vi "Test Query Parameters.vi"() -> ()   [LabVIEW 2020]
uses:
  HTTP Server/Trace Log.ctl
  HTTP Server/Trace Item.ctl
  HTTP Server/Processing Step.ctl
  <vilib>/IlluminatedG/IG HTTP Utils/HTTP Utils/Method.ctl
  TestQueryParamController/TestQueryParamController.lvclass
  C:/dev/illuminated-g/lv-http-server/HTTP Server/Handler/Handler.lvclass
  HTTP Server/Server/Add Connection Handler.vi
  HTTP Server/Server/Add Request Handler.vi
  HTTP Server/Server/Add Route Handler.vi
  HTTP Server/Server/Add Controller Handler.vi
  HTTP Server/Server/Add Controller.vi
  HTTP Server/Server/Add Response Handler.vi
  HTTP Server/Server/Add Complete Handler.vi
  HTTP Server/Server/Add Exception Handler.vi
  HTTP Server/Connection Handler/Connection Handler.lvclass
  HTTP Server/Request Handler/Request Handler.lvclass
  HTTP Server/Route Handler/Route Handler.lvclass
  HTTP Server/Controller Handler/Controller Handler.lvclass
  HTTP Server/Controller/Controller.lvclass
  HTTP Server/Response Handler/Response Handler.lvclass
  HTTP Server/Complete Handler/Complete Handler.lvclass
  HTTP Server/Exception Handler/Exception Handler.lvclass
  HTTP Server/Server/Server.lvclass
  HTTP Server/Handler/Handler.lvclass
  HTTP Server/RequestTraceLog/RequestTraceLog.lvclass
  HTTP Server/HTTP Server.lvlib
  <vilib>/IlluminatedG/IG HTTP Utils/HTTP Utils/HTTP Utils.lvlib
panel:
  out "error out":errorcluster
  in  "Refresh Traces":bool
  out "Traces":T1[](array[typedef])=[{"Items"=[{"Duration"=0.00019280000014987309, "Step"=enum."Connection", "Class"="", "Info"="Start Request Parsing", "Status"=FALSE, "Code"=0, "Time"=3234.2736639}, {"Duration"=104.21120999999994, "Step"=enum."Connection", "Class"="", "Info"="Request Initialized", "Status"=TRUE, "Code"=66, "Time"=3338.4848739}, {"Duration"=0.0007422999997288571, "Step"=enum."Connection", "Class"="HTTP Utils.lvlib:Response.lvclass", "Info"="Completed", "Status"=TRUE, "Code"=66, "Time"=3338.4856161999996}], "Client"="tcp://DAB-2020SP1x86.ni.corp.natinst.com:52788", "Target"="", "Response Type"="", "Processing"=0.0007728000000497559, "Status"=200, "Method"=enum."GET", "Content Type"="", "Request Headers"=[], "Parsing"=3338.4848739, "Waiting"=-3234.2736639, "Identity"="", "Loaded"=FALSE, "Created"=FALSE, "Destroyed"=FALSE, "Response Headers"=[], "Created"=0.0, "Expires"=0.0, "Roles"=[], "Sending"=0.0}, {"Items"=[{"Duration"=0.006463199999870994, "Step"=enum."Connection", "Class"="", "Info"="Start Request Parsing", "Status"=FALSE, "Code"=0, "Time"=3459.3199179}, {"Duration"=0.008297200000015437, "Step"=enum."Connection", "Class"="", "Info"="Request Initialized", "Status"=TRUE, "Code"=66, "Time"=3459.3282151}, {"Duration"=0.0001554000000396627, "Step"=enum."Connection", "Class"="HTTP Utils.lvlib:Response.lvclass", "Info"="Completed", "Status"=TRUE, "Code"=66, "Time"=3459.3283705}], "Client"="tcp://DAB-2020SP1x86.ni.corp.natinst.com:52995", "Target"="", "Response Type"="", "Processing"=0.00019930000007661874, "Status"=200, "Method"=enum."GET", "Content Type"="", "Request Headers"=[], "Parsing"=3459.3282151, "Waiting"=-3459.3199179, "Identity"="", "Loaded"=FALSE, "Created"=FALSE, "Destroyed"=FALSE, "Response Headers"=[], "Created"=0.0, "Expires"=0.0, "Roles"=[], "Sending"=0.0}] {"Sending" format="%_6f"; "Expires" format="%<%X %x>T"; "Created" format="%<%X %x>T"; "Waiting" format="%_6f"; "Parsing" format="%_6f"; "Processing" format="%_6f"; "Items"."Time" format="%.6f"; "Items"."Duration" format="%.6f"}
  in  "Port":u16=36987
  # "This can be viewed at http://localhost:36987/calc and filling out the query parameters as specified in the page.\n\nRequests to any other path will result in a 404 status."
  # "Request"
  # "Response"
  # "Session"
  # "Auth"
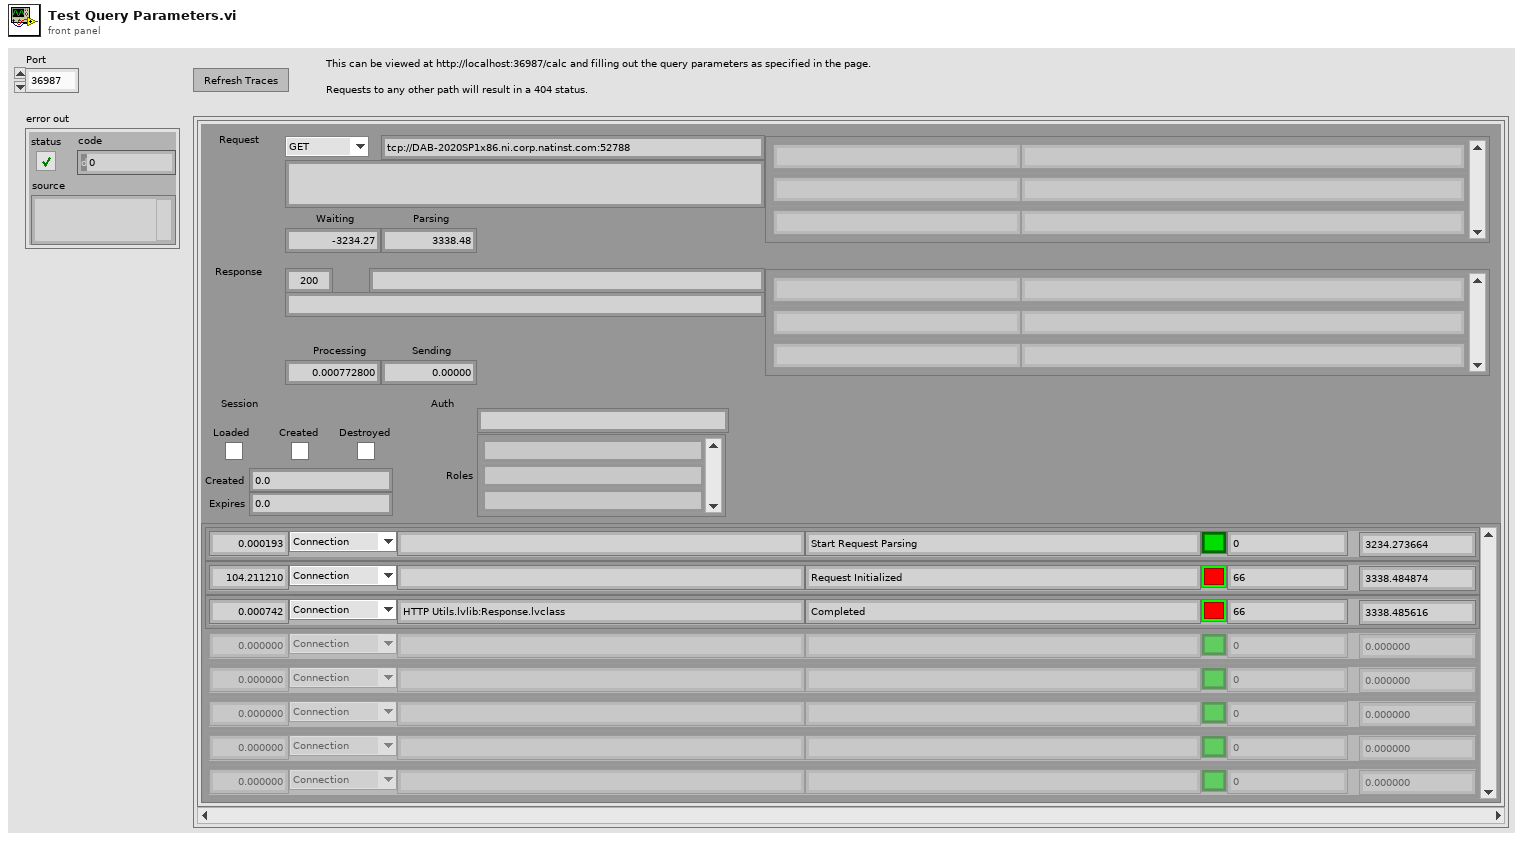
[diagram p1: front panel]
types:
  T1 = typedef "HTTP Server.lvlib/Trace Log.ctl" = cluster{"Items":T2[], "Client":string, "Target":string, "Response Type":string, "Processing":dbl, "Status":u16, "Method":T4, "Content Type":string, "Request Headers":cluster{"Name":string, "Value":string}[], "Parsing":dbl, "Waiting":dbl, "Identity":string, "Loaded":bool, "Created":bool, "Destroyed":bool, "Response Headers":cluster{"Name":string, "Value":string}[], "Created":dbl, "Expires":dbl, "Roles":string[], "Sending":dbl}
  T2 = typedef "HTTP Server.lvlib/Trace Item.ctl" = cluster{"Duration":dbl, "Step":T3, "Class":string, "Info":string, "Status":bool, "Code":i32, "Time":dbl}
  T3 = typedef "HTTP Server.lvlib/Processing Step.ctl" = enum16{"Connection", "Request", "Routing", "Controller Init", "Controller", "Response", "Complete", "Exception"}
  T4 = typedef "HTTP Utils.lvlib/Method.ctl" = enum16{"GET", "HEAD", "POST", "PUT", "DELETE", "CONNECT", "OPTIONS", "TRACE", "PATCH"}
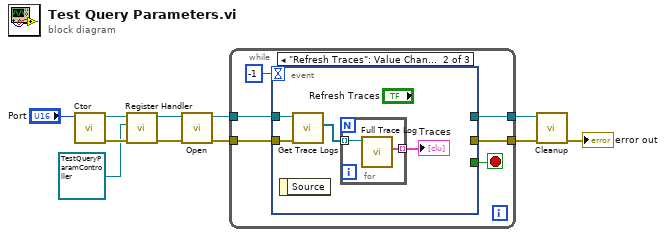
[diagram p0: block diagram]
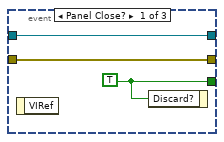
[diagram p2: hidden frame]
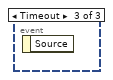
[diagram p3: hidden frame]
diagram:
  n1 = call "Ctor.vi"("HTTP Port (80)"="Port") -> ("error out"=w3:errorcluster, "Server out"=w6:refnum<class "Server.lvclass">)  [unwired: 9 in]
  n2 = call "Register Handler.vi"("error in (no error)"=w3, "Handler"=refnum<class "TestQueryParamController.lvclass"> refnum ("TestQueryParamController.lvclass"), "Server in"=w6) -> ("error out"=w4:errorcluster, "Server out"=w5:refnum<class "Server.lvclass">)  [unwired: 7 in]
  n3 = call "Open.vi"("error in (no error)"=w4, "Server in"=w5) -> ("error out"=w9:errorcluster, "Server out"=w10:refnum<class "Server.lvclass">)  [unwired: 8 in]
  n4 = while {
    tunnel: w10 -> [w15]
    tunnel: w9 -> [w16]
    tunnel: [w14] -> w8
    tunnel: [w13] -> w7
    stop <- w17 stop-if-true
    n5 = event shown="[1] \"Refresh Traces\": Value Change" {
      selector: _ -> [_ _ _]
      dyn-events: _ -> [_ _ _]
      timeout: -1 -> [_ _ _]
      tunnel: [w20 _ _] -> w17
      tunnel: w16 -> [w18 w22 _]
      tunnel: w15 -> [w19 w23 _]
      tunnel: [w19 _ _] -> w14
      tunnel: [w18 _ _] -> w13
      event Panel Close? {
        w20 = TRUE ("Discard?")
        n6 = event-data() -> ()  [unwired: 1 in, 1 out]
        n7 = event-data("Discard?"=w20) -> ()  [unwired: 1 in, 1 out]
      }
      event "Refresh Traces": Value Change {
        n8 = event-data() -> ()  [unwired: 1 in, 1 out]
        n9 = call "Get Trace Logs.vi"("error in (no error)"=w22, "Server in"=w23) -> ("Trace Logs"=w24:refnum<class "RequestTraceLog.lvclass">[])  [unwired: 7 in, 2 out]
        n10 = for {
          tunnel: w24 -> [w26] mode=indexing
          tunnel: [w25] -> w21 mode=indexing
          n11 = call "Full Trace Log.vi"("RequestTraceLog in"=w26) -> ("Trace Log"=w25:T1)  [unwired: 8 in, 2 out]
        }
        "Traces" <- w21
      }
      event Timeout {
        n12 = event-data() -> ()  [unwired: 1 in, 1 out]
      }
    }
  }
  n13 = call "Cleanup.vi"("error in (no error)"=w7, "Server in"=w8) -> ("error out"=→"error out":errorcluster)  [unwired: 9 in]
